vi "specrugram.vi"(10 "Numeric":ext, 11 "Array in":cdb[](array[numeric])) -> (3 "Array out":dbl[][](array[numeric]))   [LabVIEW 2021]
uses:
  <vilib>/measure/NI_MAPro.lvlib
  <vilib>/measure/maspectr.llb/FFT Power Spectrum and PSD for 1 Chan (CDB).vi
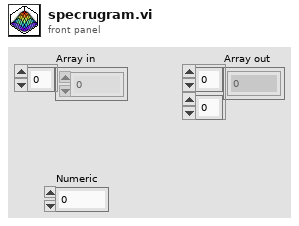
[diagram p1: front panel]
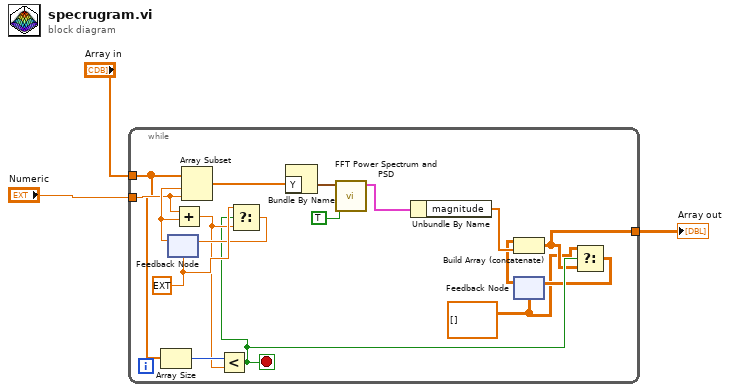
[diagram p0: block diagram]
diagram:
  n1 = while {
    tunnel: "Numeric" -> [w13]
    tunnel: [w5] -> w2
    tunnel: "Array in" -> [w11]
    stop <- w7 stop-if-true
    w4 = dbl[][] []
    w10 = ext 0.0 ("x")
    n2 = Array Size(array=w11) -> (size(s)=w18:i32)
    n3 = feedback #1(w10) -> (w14:ext)
    n4 = Add(x=w13, y=w14) -> (x+y=w8:ext)
    n5 = Array Subset(array=w11, index=w14, length=w13) -> (w12:cdb[])
    n6 = Less?(x=w18, y=w8) -> (x < y?=w7:bool)
    n7 = Select(t=w10, s=w7, f=w8) -> (s? t:f=w9:ext)
    n8 = feedback-in #1(w9) -> ()
    n9 = Bundle By Name("Y"=w12) -> (w20:waveform(cdb))  [unwired: 1 in]
    n10 = call-poly <vilib>:"FFT Power Spectrum and PSD.vi"("dB On (F)"=TRUE, "time signal"=w20) -> ("Power Spectrum / PSD"=w17:cluster{"f0":dbl, "df":dbl, "magnitude":dbl[]})  [unwired: 6 in, 3 out]
    n11 = Unbundle By Name(w17) -> ("magnitude"=w16:dbl[])
    n12 = feedback #2(w4) -> (w15:dbl[][])
    n13 = Build Array (concatenate)(w15, w16) -> (w5:dbl[][])
    n14 = Select(t=w4, s=w7, f=w5) -> (s? t:f=w6:dbl[][])
    n15 = feedback-in #2(w6) -> ()
  }
  "Array out" <- w2
